vi "PDF_Bold-Normal_line.vi"(5 "Bold header":string, 7 "Normal text":string, 8 "error in (no error)":errorcluster, 11 "PDF Report IN":T21(xcontrol)) -> (0 "error out":errorcluster, 3 "PDF Report duplicate":T21(xcontrol))   [LabVIEW 2013]
uses:
  Utils/Exaprom PDF/Controls/PDF Report Xcontrol/PDF Report.xctl
  Utils/Exaprom PDF/VIs/Text/Append Phrase.vi
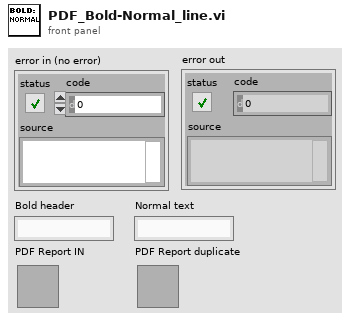
[diagram p1: front panel]
types:
  T1 = typedef "Font cluster.ctl" = cluster{"Name":string, "Size":T2, "Color":T3, "Style":cluster{"Bold":bool, "Italic":bool, "Underline":bool, "Strikeout":bool}}
  T2 = typedef "Font size.ctl" = sgl
  T3 = typedef "Font color.ctl" = u32
  T4 = typedef "Unit.ctl" = enum16{"inch", "mm"}
  T5 = typedef "Paragraphe cluster.ctl" = cluster{" Aligment":T6, "Line spacing":T7}
  T6 = typedef "Texte alignement.ctl" = enum16{"Select", "CENTER", "JUSTIFY", "LEFT", "RIGHT"}
  T7 = typedef "Line spacing.ctl" = enum16{"Select", "1.0", "1.5", "2.0"}
  T8 = typedef "Page dimensions.ctl" = cluster{"Start at page":i32, "Orientation":T9, "widht":sgl, "height":sgl, "Margin left":sgl, "Margin right":sgl, "Margin top":sgl, "Margin bottom":sgl}
  T9 = typedef "Page Orientation.ctl" = enum16{"Portrait", "Landscape"}
  T10 = typedef "Image or Table Caption.ctl" = cluster{"Caption":string, "Separator":string, "Position":enum16{"Above", "Below"}}
  T11 = typedef "Header Footer [ ].ctl" = T12[]
  T12 = typedef "Header Footer cluster.ctl" = cluster{"Start page":i32, "Type":T13, "Alignment":T14, "Vertical Alignement":T15, "Image (%)":sgl, "Page #":T16, "Text":string, "Path":string, "Font":T1, "Font refnum":refnum<k24>, "Line":cluster{"Line":T17, "Thickness (points)":sgl, "Colour":T3}}
  T13 = typedef "Header Footer Type.ctl" = enum16{"Select", "Text", "Text + hyperlink", "Page number", "Image", "Image + hyperlink"}
  T14 = typedef "Header footer horiz alignment.ctl" = enum16{"Left", "Center", "Right"}
  T15 = typedef "Cell Vertical alignment.ctl" = enum16{"TOP", "MIDDLE", "BOTTOM"}
  T16 = typedef "Page number.ctl" = cluster{"Text 1":string, "Text 2":string, "Text 3":string}
  T17 = typedef "Header Footer Line.ctl" = enum16{"No line", "Horizontal line"}
  T18 = typedef "Watermark cluster2.ctl" = cluster{"Show? (F)":bool, "Type":enum16{"Image", "Text"}, "Opacity (%)":sgl, "Rotate(°)":sgl, "Position":cluster{"Position":T19, "X":sgl, "Y":sgl}, "Image path":path, "Scaled(%)":sgl, "Image refnum":refnum<k24>, "Text":string, "Font":cluster{"Name":string, "Size":T2, "Color":T3}, "Font refnum":refnum<k24>, "Alignment":T14, "Automatic":bool}
  T19 = typedef "Watermark Position.ctl" = enum16{"Absolute", "Center (page)", "Center (text section)"}
  T20 = typedef "System Fonts.ctl" = cluster{"Font name [ ]":string[], "Font and file names [ ]":cluster{"Font name":string, "File name":string}[]}
  T21 = cluster{"Document":refnum<k24>, "Writer":refnum<k24>, "Default Font":refnum<k24>, "Default Font cluster":T1, "Path":path, "Unit (default = mm)":T4, "Paragraphe cluster":T5, "Pages dimensions [ ]":T8[], "Captions":cluster{"Image":T10, "Image counter":u16, "Table":T10, "Table counter":u16, "Font":T1}, "Header":T11, "Footer":T11, "Watermark ":T18, "Actual VI name":string, "System Fonts":T20}
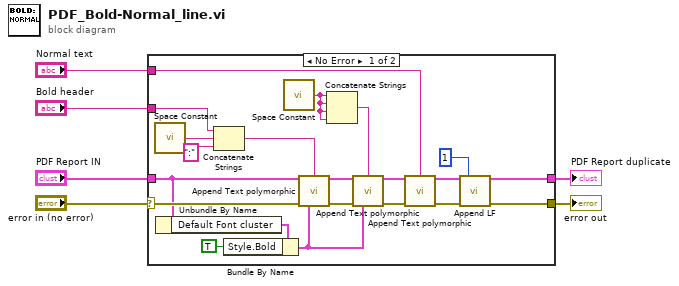
[diagram p0: block diagram]
diagram:
  n1 = case shown="No Error" "error in (no error)" {
    selector: "error in (no error)" -> [w24 w29]
    tunnel: [w23 w29] -> w5
    tunnel: [w22 w28] -> w4
    tunnel: "PDF Report IN" -> [w10 w28]
    tunnel: "Bold header" -> [w20 _]
    tunnel: "Normal text" -> [w19 _]
    frame No Error {
      n2 = call <vilib>:"Space Constant.vi"() -> ("String"=w11:string)
      n3 = Unbundle By Name(w10) -> ("Default Font cluster"=w9:T1)
      n4 = Concatenate Strings(w20, w11, ":") -> (w21:string)
      n5 = Bundle By Name(cluster=w9, "Style.Bold"=TRUE) -> (w8:T1)
      n6 = call <vilib>:"Space Constant.vi"() -> ("String"=w13:string)
      n7 = call-poly "Append Text polymorphic.vi"("PDF Report IN"=w10, "Text"=w21, "error in (no error)"=w24, "Font"=w8) -> ("PDF Report OUT"=w18:T21, "error out"=w17:errorcluster)  [unwired: 10 in]
      n8 = Concatenate Strings(w13, w13, w13, w13) -> (w14:string)
      n9 = call-poly "Append Text polymorphic.vi"("PDF Report IN"=w18, "Text"=w14, "error in (no error)"=w17, "Font"=w8) -> ("PDF Report OUT"=w16:T21, "error out"=w15:errorcluster)  [unwired: 10 in]
      n10 = call-poly "Append Text polymorphic.vi"("PDF Report IN"=w16, "Text"=w19, "error in (no error)"=w15) -> ("PDF Report OUT"=w27:T21, "error out"=w26:errorcluster)  [unwired: 11 in]
      n11 = call "Append LF.vi"("PDF Report IN"=w27, "Number of LF (default 1)"=1, "error in (no error)"=w26) -> ("PDF Report duplicate"=w22:T21, "error out"=w23:errorcluster)  [unwired: 11 in]
    }
    frame Error {
    }
  }
  "error out" <- w5
  "PDF Report duplicate" <- w4
